vi "New DBL Pointer.vi"(8 "error in (no error)":errorcluster, 11 "channel count":u64) -> (0 "error out":errorcluster, 3 "DBL Pointer out":refnum<class "DBL Pointer.lvclass">)   [LabVIEW 2017, in "DSF Core.lvlib" / "DBL Pointer.lvclass"]
uses:
  DBL Pointer.lvclass
  DBL Pointer.lvclass/DBL Pointer.ctl
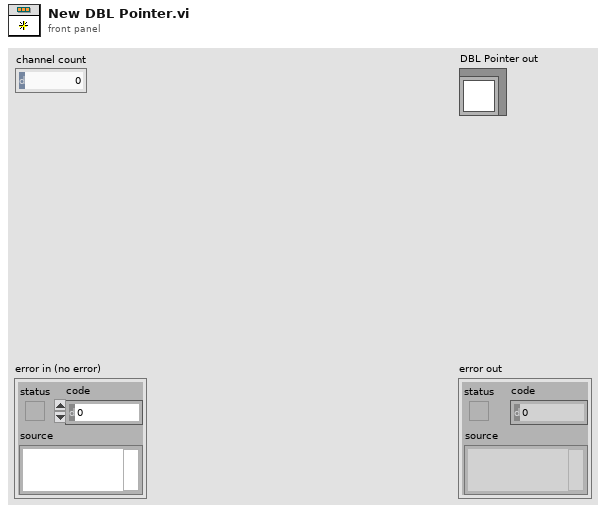
[diagram p1: front panel]
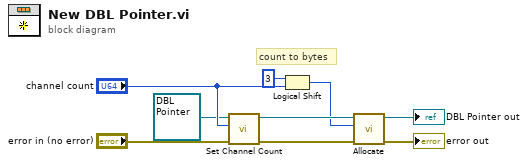
[diagram p0: block diagram]
diagram:
  # "count to bytes"
  n1 = call "Set Channel Count.vi"("channel count"="channel count", "DBL Buffer in"=refnum<class "DBL Pointer.lvclass"> refnum) -> ("DBL Buffer out"=w8:refnum<class "DBL Pointer.lvclass">)  [unwired: 9 in]
  n2 = Logical Shift(y=i16 3, x="channel count") -> (x << y=w2:u64)
  n3 = call-dynamic "Allocate.vi"("error in (no error)"="error in (no error)", "size"=w2, "Pointer in"=w8) -> ("error out"=→"error out":errorcluster, "Pointer out"=→"DBL Pointer out":refnum<class "DBL Pointer.lvclass">)  [unwired: 7 in]
